vi "del-exp-eventSD.vi"(1 "cluster in":T1={"Kinetics"=[], "Spectrum"=[], "Experiments groups"=[], "GRAPH EXPERIMENTAL DATA"=[], "error out"={"status"=FALSE, "code"=0, "source"=""}, "group"=0, "exp selected"=0, "# exp"=0, "kinetics plot names"=[], "spectra plot names"=[], "FromToWave"={"FromWave"=0.0, "ToWave"=0.0}, "Laser shutter task"="", "Accelerator task"="", "Motor task"="", "GRAPH EXPERIMENTAL DATA ref"=refnum, "timedelays"=[0.0, 0.0, 0.0, 0.0, 0.0, 0.0, 0.0, 0.06019061100911815, 0.0521779104562645, 0.045231877429679615, 0.03921051490799832, 0.033990728811568754, 0.029465811603150715, 0.025543260876973825, 0.02214288834180205, 0.01919518054014414, 0.016639877791965713, 0.014424742312398925, 0.012504490320209958, 0.010839866306230088, 0.009396840537117498, 0.008145913389103785, 0.00706151229029317, 0.006121468943269439, 0.005306566140927374, 0.004600144911132549, 0.003987763959109073, 0.0034569044455719407, 0.00299671406541447, 0.0025977851951783253, 0.0022519625739982996, 0.00195217658646366, 0.0016922987392150965, 0.0014670163768006634, 0.0012717240756200802, 0.0011024294957352762, 0.0009556717658856477, 0.0008284507332614981, 0.0007181656316962257, 0.0006225619144775864, 0.0005396851648867825, 0.00046784114226338394, 0.0004055611468220084, 0.0003515719951773376, 0.00030476999279031153, 0.00026419837125694315, 0.00022902772919263772, 0.0001985390768670671, 0.0001721091379728629, 0.00014919760805372974, 0.00012933610911736794], "wavelengths"=[0.0, 0.0, 0.0, 0.0, 0.0, 0.0, 0.0, 0.06019061100911815, 0.0521779104562645, 0.045231877429679615, 0.03921051490799832, 0.033990728811568754, 0.029465811603150715, 0.025543260876973825, 0.02214288834180205, 0.01919518054014414, 0.016639877791965713, 0.014424742312398925, 0.012504490320209958, 0.010839866306230088, 0.009396840537117498, 0.008145913389103785, 0.00706151229029317, 0.006121468943269439, 0.005306566140927374, 0.004600144911132549, 0.003987763959109073, 0.0034569044455719407, 0.00299671406541447, 0.0025977851951783253, 0.0022519625739982996, 0.00195217658646366, 0.0016922987392150965, 0.0014670163768006634, 0.0012717240756200802, 0.0011024294957352762, 0.0009556717658856477, 0.0008284507332614981, 0.0007181656316962257, 0.0006225619144775864, 0.0005396851648867825, 0.00046784114226338394, 0.0004055611468220084, 0.0003515719951773376, 0.00030476999279031153, 0.00026419837125694315, 0.00022902772919263772, 0.0001985390768670671, 0.0001721091379728629, 0.00014919760805372974, 0.00012933610911736794], "Experiment"=refnum, "Commentaires exp"=refnum, "FromToDelay"={"FromDelay"=0.0, "ToDelay"=0.0}}, 2 "Update graphs of exp":refnum<user-event>) -> (0 "cluster out":T1={"Kinetics"=[], "Spectrum"=[], "Experiments groups"=[], "GRAPH EXPERIMENTAL DATA"=[], "error out"={"status"=FALSE, "code"=0, "source"=""}, "group"=0, "exp selected"=0, "# exp"=0, "kinetics plot names"=[], "spectra plot names"=[], "FromToWave"={"FromWave"=0.0, "ToWave"=0.0}, "Laser shutter task"="", "Accelerator task"="", "Motor task"="", "GRAPH EXPERIMENTAL DATA ref"=refnum, "timedelays"=[0.0, 0.0, 0.0, 0.0, 0.0, 0.0, 0.0, 0.06019061100911815, 0.0521779104562645, 0.045231877429679615, 0.03921051490799832, 0.033990728811568754, 0.029465811603150715, 0.025543260876973825, 0.02214288834180205, 0.01919518054014414, 0.016639877791965713, 0.014424742312398925, 0.012504490320209958, 0.010839866306230088, 0.009396840537117498, 0.008145913389103785, 0.00706151229029317, 0.006121468943269439, 0.005306566140927374, 0.004600144911132549, 0.003987763959109073, 0.0034569044455719407, 0.00299671406541447, 0.0025977851951783253, 0.0022519625739982996, 0.00195217658646366, 0.0016922987392150965, 0.0014670163768006634, 0.0012717240756200802, 0.0011024294957352762, 0.0009556717658856477, 0.0008284507332614981, 0.0007181656316962257, 0.0006225619144775864, 0.0005396851648867825, 0.00046784114226338394, 0.0004055611468220084, 0.0003515719951773376, 0.00030476999279031153, 0.00026419837125694315, 0.00022902772919263772, 0.0001985390768670671, 0.0001721091379728629, 0.00014919760805372974, 0.00012933610911736794], "wavelengths"=[0.0, 0.0, 0.0, 0.0, 0.0, 0.0, 0.0, 0.06019061100911815, 0.0521779104562645, 0.045231877429679615, 0.03921051490799832, 0.033990728811568754, 0.029465811603150715, 0.025543260876973825, 0.02214288834180205, 0.01919518054014414, 0.016639877791965713, 0.014424742312398925, 0.012504490320209958, 0.010839866306230088, 0.009396840537117498, 0.008145913389103785, 0.00706151229029317, 0.006121468943269439, 0.005306566140927374, 0.004600144911132549, 0.003987763959109073, 0.0034569044455719407, 0.00299671406541447, 0.0025977851951783253, 0.0022519625739982996, 0.00195217658646366, 0.0016922987392150965, 0.0014670163768006634, 0.0012717240756200802, 0.0011024294957352762, 0.0009556717658856477, 0.0008284507332614981, 0.0007181656316962257, 0.0006225619144775864, 0.0005396851648867825, 0.00046784114226338394, 0.0004055611468220084, 0.0003515719951773376, 0.00030476999279031153, 0.00026419837125694315, 0.00022902772919263772, 0.0001985390768670671, 0.0001721091379728629, 0.00014919760805372974, 0.00012933610911736794], "Experiment"=refnum, "Commentaires exp"=refnum, "FromToDelay"={"FromDelay"=0.0, "ToDelay"=0.0}})   [LabVIEW 2015]
uses:
  controls/control-cluster.ctl
  Classes/Experiments_group.lvclass
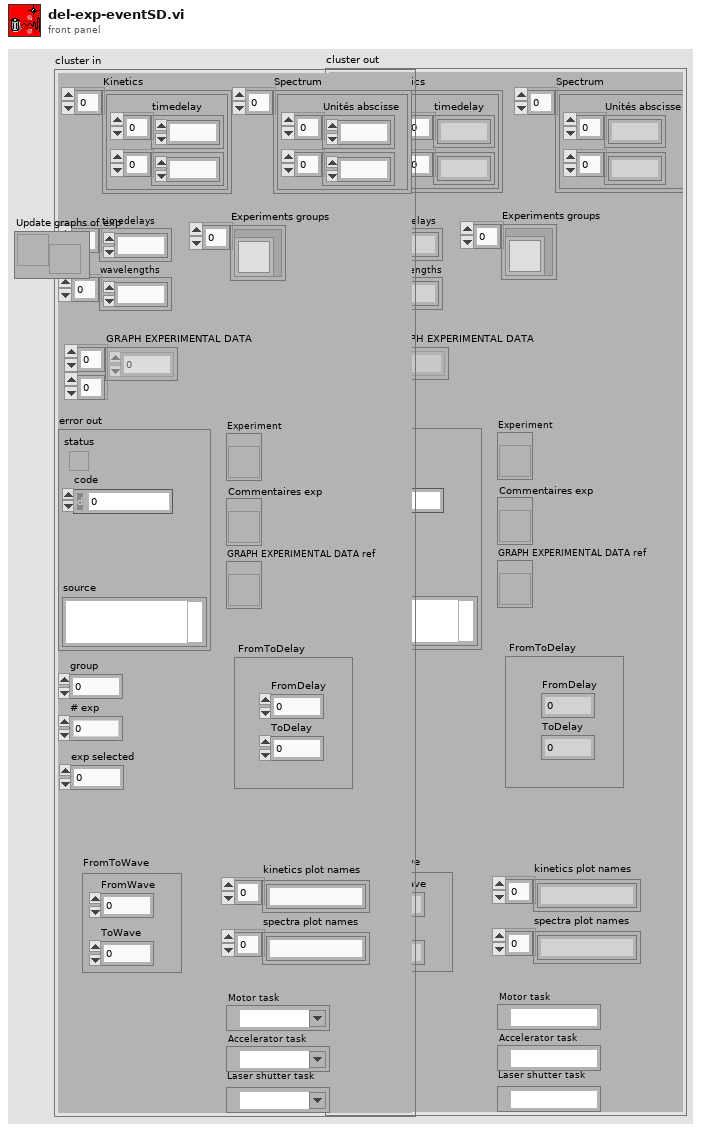
[diagram p1: front panel]
types:
  T1 = typedef "control-cluster.ctl" = cluster{"Kinetics":cluster{"timedelay":dbl[], dbl[]}[], "Spectrum":cluster{"Unités abscisse":dbl[], dbl[]}[], "Experiments groups":refnum<class "Experiments_group.lvclass">[], "GRAPH EXPERIMENTAL DATA":dbl[][], "error out":errorcluster, "group":i32, "exp selected":i32, "# exp":i32, "kinetics plot names":string[], "spectra plot names":string[], "FromToWave":cluster{"FromWave":dbl, "ToWave":dbl}, "Laser shutter task":refnum<k21>, "Accelerator task":refnum<k21>, "Motor task":refnum<k21>, "GRAPH EXPERIMENTAL DATA ref":refnum<vi>, "timedelays":dbl[], "wavelengths":dbl[], "Experiment":refnum<vi>, "Commentaires exp":refnum<vi>, "FromToDelay":cluster{"FromDelay":dbl, "ToDelay":dbl}}
  T2 = cluster{bool, "Item Names":string[], "exp selected":i32}
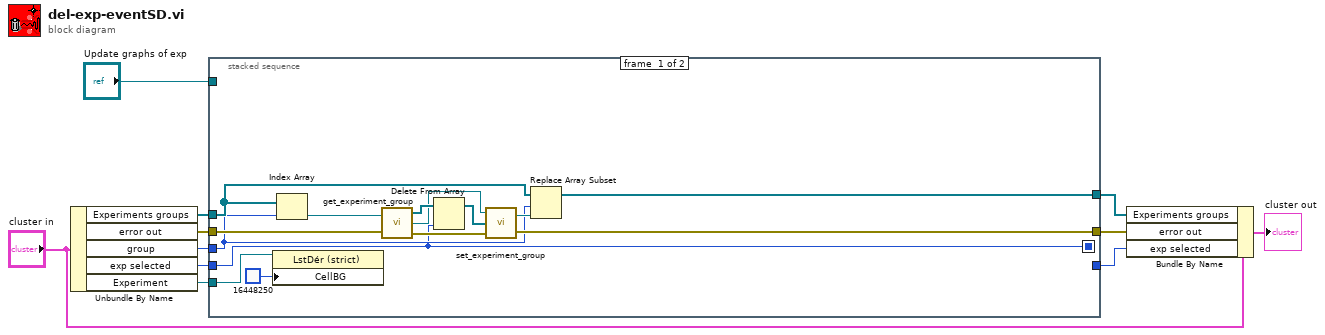
[diagram p0: block diagram]
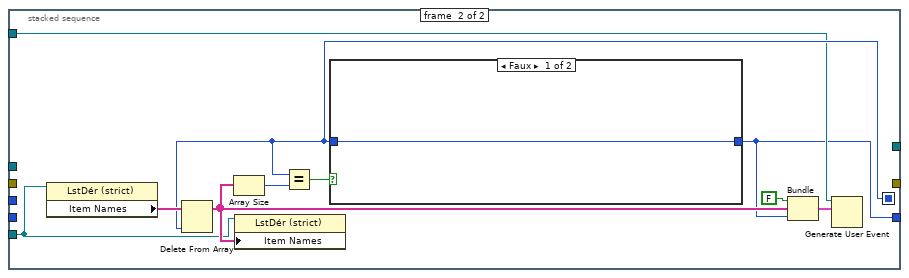
[diagram p2: hidden frame]
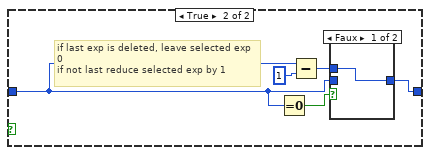
[diagram p3: hidden frame]
diagram:
  n1 = Unbundle By Name("cluster in") -> ("Experiments groups"=w8:refnum<class "Experiments_group.lvclass">[], "error out"=w7:errorcluster, "group"=w4:i32, "exp selected"=w3:i32, "Experiment"=w1:refnum<vi>)
  n2 = stacked-sequence {
    seq-local: [w13 _] -> [_ w29]
    tunnel: [w20 _] -> w5
    tunnel: [w19 _] -> w6
    tunnel: "Update graphs of exp" -> [_ w28]
    tunnel: w8 -> [w15 _]
    tunnel: w7 -> [w17 _]
    tunnel: w4 -> [w14 _]
    tunnel: w3 -> [w13 _]
    tunnel: [_ w27] -> w2
    tunnel: w1 -> [w12 w26]
    frame #0 {
      n3 = property on="Property Node" class="LstDér (strict)"(reference=w12, "CellBG"=u32 16448250) -> ()  [unwired: 1 in, 2 out]
      n4 = Index Array(array=w15, index=w14) -> (element=w16:refnum<class "Experiments_group.lvclass">)
      n5 = call-dynamic "get_experiment_group.vi"("Experiments_group.lvclass in"=w16, "error in (no error)"=w17) -> ("Experiments"=w25:refnum<class "Experiment.lvclass">[], "Experiments_group.lvclass out"=w24:refnum<class "Experiments_group.lvclass">, "error out"=w22:errorcluster)
      n6 = Delete From Array(array=w25, index=w13) -> (array with subset deleted=w21:refnum<class "Experiment.lvclass">[])  [unwired: 1 in, 1 out]
      n7 = call-dynamic "set_experiment_group.vi"("error in (no error)"=w22, "Experiments"=w21, "Experiments_group.lvclass in"=w24) -> ("error out"=w19:errorcluster, "Experiments_group.lvclass out"=w23:refnum<class "Experiments_group.lvclass">)
      n8 = Replace Array Subset(array=w15, new element=w23, index=w14) -> (w20:refnum<class "Experiments_group.lvclass">[])
    }
    frame #1 {
      n9 = property on="Property Node" class="LstDér (strict)"(reference=w26) -> ("Item Names"=w32:string[])  [unwired: 1 in, 2 out]
      n10 = Delete From Array(array=w32, index=w29) -> (array with subset deleted=w31:string[])  [unwired: 1 in, 1 out]
      n11 = Array Size(array=w31) -> (size(s)=w30:i32)
      n12 = property on="Property Node" class="LstDér (strict)"(reference=w26, "Item Names"=w31) -> ()  [unwired: 1 in, 2 out]
      n13 = Equal?(x=w29, y=w30) -> (x = y?=w33:bool)
      n14 = case shown="Faux" w33 {
        tunnel: w29 -> [w36 w39]
        tunnel: [w36 w38] -> w27
        frame False {
        }
        frame True {
          # "if last exp is deleted, leave selected exp\n0\nif not last reduce selected exp by 1"
          n15 = Equal To 0?(x=w39) -> (x = 0?=w40:bool)
          n16 = Subtract(x=w39, y=1) -> (x-y=w37:i32)
          n17 = case shown="Faux" w40 {
            tunnel: [w42 w43] -> w38
            tunnel: w39 -> [_ w43]
            tunnel: w37 -> [w42 _]
            frame False {
            }
            frame True {
            }
          }
        }
      }
      n18 = Bundle(FALSE, "Item Names"=w31, "exp selected"=w27) -> (w34:T2)  [unwired: 1 in]
      n19 = Generate User Event(user event=w28, event data cluster=w34) -> ()  [unwired: 2 in, 2 out]
    }
  }
  n20 = Bundle By Name(cluster="cluster in", "Experiments groups"=w5, "error out"=w6, "exp selected"=w2) -> (→"cluster out":T1)
